vi "04TRM800_AnalyzeReceive.vi"(8 "error in (no error)":errorcluster, 10 "String":string, 11 "Enum":enum16{"Initialize", "Analyze"}(ring)) -> (0 "error out":errorcluster)   [LabVIEW 2020]
uses:
  <vilib>/regexp/Match Regular Expression.xnode
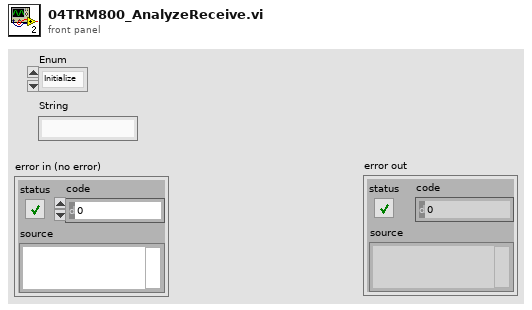
[diagram p1: front panel]
types:
  T1 = enum16{"Initialize", "Next", "SendRSET", "SetMPH", "SetINC"}
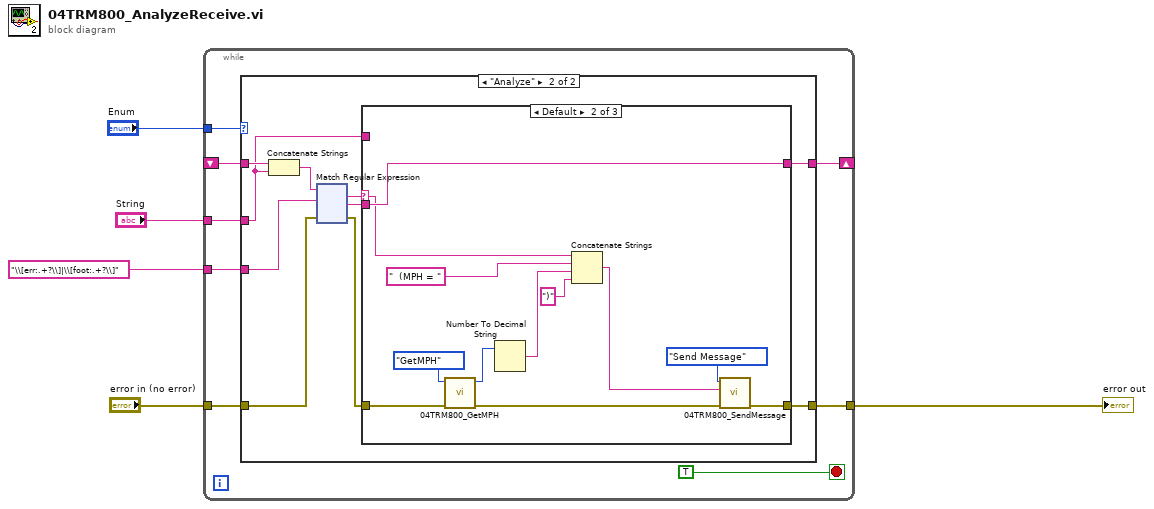
[diagram p0: block diagram]
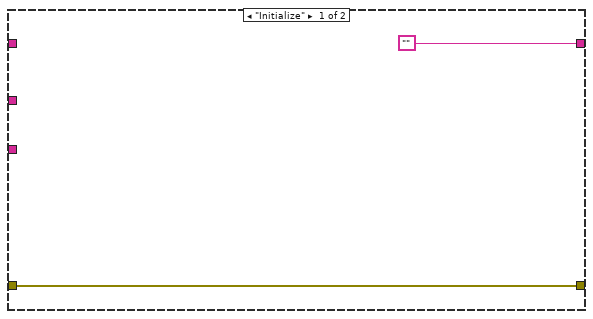
[diagram p2: hidden frame]
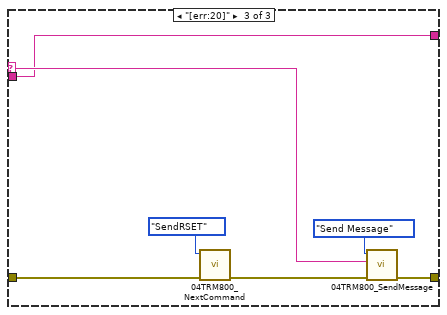
[diagram p4: hidden frame]
diagram:
  n1 = while {
    tunnel: "error in (no error)" -> [w10]
    tunnel: [w11] -> w4
    tunnel: "Enum" -> [w12]
    shift-right: [w9] -> _
    shift-left: _ -> [w8]
    tunnel: "String" -> [w7]
    tunnel: "\\[err:.+?\\]|\\[foot:.+?\\]" ("regular expression") -> [w6]
    stop <- TRUE stop-if-true
    n2 = case shown="\"Analyze\"" w12 {
      tunnel: [w15 w20] -> w11
      tunnel: w10 -> [w15 w17]
      tunnel: ["" w22] -> w9
      tunnel: w8 -> [_ w25]
      tunnel: w7 -> [_ w23]
      tunnel: w6 -> [_ w19]
      frame "Initialize" {
      }
      frame "Analyze" {
        n3 = Concatenate Strings(w25, w23) -> (w18:string)
        n4 = xnode "Match Regular Expression"("input string"=w18, "regular expression"=w19, "error in"=w17) -> ("whole match"=w24:string, "after match"=w21:string, "error out"=w16:errorcluster)  [unwired: 3 in, 2 out]
        n5 = case shown="Default" w24 {
          selector: w24 -> [_ w146 w158]
          tunnel: w23 -> [w141 _ _]
          tunnel: [w141 w151 w157] -> w22
          tunnel: w21 -> [_ w151 w157]
          tunnel: [w140 w152 w159] -> w20
          tunnel: w16 -> [w140 w150 w155]
          frame "" {
          }
          frame Default {
            n6 = call "04TRM800_GetMPH.vi"("error in (no error)"=w150, "Initialize"=enum16{"Initialize", "GetMPH"}."GetMPH") -> ("error out"=w149:errorcluster, "MPH"=w147:i32)  [unwired: 8 in]
            n7 = Number To Decimal String(number=w147) -> (decimal integer string=w144:string)  [unwired: 1 in]
            n8 = Concatenate Strings(w146, "  (MPH = " ("string"), w144, ")" ("string")) -> (w142:string)
            n9 = call "04TRM800_SendMessage.vi"("error in (no error)"=w149, "String"=w142, "Enum"=enum16{"Initialize", "Send Message"}."Send Message") -> ("error out"=w152:errorcluster)  [unwired: 8 in]
          }
          frame "[err:20]" {
            n10 = call "04TRM800_NextCommand.vi"("error in (no error)"=w155, "Enum"=T1."SendRSET") -> ("error out"=w154:errorcluster)  [unwired: 8 in, 1 out]
            n11 = call "04TRM800_SendMessage.vi"("error in (no error)"=w154, "String"=w158, "Enum"=enum16{"Initialize", "Send Message"}."Send Message") -> ("error out"=w159:errorcluster)  [unwired: 8 in]
          }
        }
      }
    }
  }
  "error out" <- w4
